vi "Retrieve Root Actor.vi"(8 "error in (no error)":errorcluster, 11 "Target Store in":refnum<class "Live Store.lvclass">) -> (0 "error out":errorcluster, 1 "valid?":bool, 2 "Root Actor":path, 3 "Target Store out":refnum<class "Live Store.lvclass">)   [LabVIEW 2023, in "Add Async Methods Actor.lvlib" / "Live Store.lvclass"]
uses:
  Live Store.lvclass
  Live Store.lvclass/Live Store.ctl
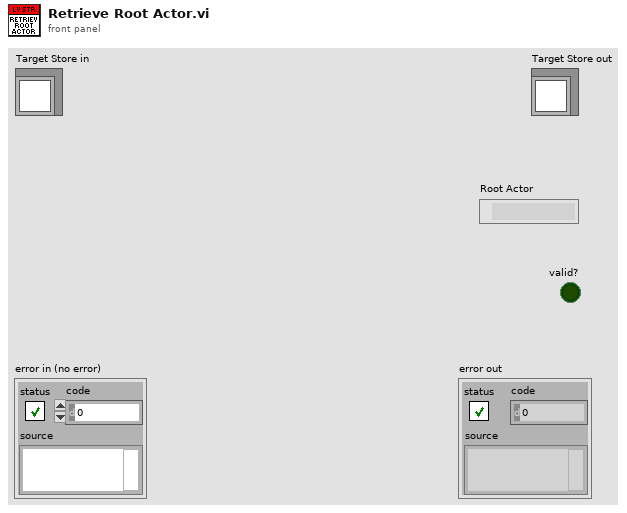
[diagram p1: front panel]
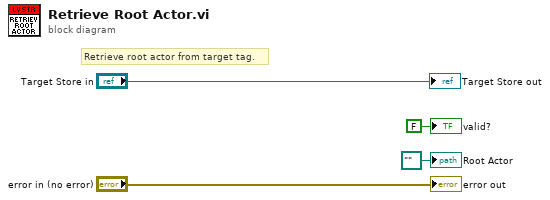
[diagram p0: block diagram]
diagram:
  # "Retrieve root actor from target tag."
  "error out" <- "error in (no error)"
  "Root Actor" <- path "" ("Root Actor")
  "valid?" <- FALSE ("valid?")
  "Target Store out" <- "Target Store in"
